vi "Driver - DTACQ - Get Detailed List of Commands.vi"(8 "error in":errorcluster, 11 "DTACQ Connection Data In":T1={"Description"="", "Address"="", "Port"=0, "timeout (ms)"=5000, "Termination Character"="\n", "TCP Connection Reference"=refnum, "Open Connection"=FALSE}) -> (0 "error out":errorcluster, 1 "Write Access":bool[](array[boolean]), 2 "Read Access":bool[](array[boolean]), 3 "DTACQ Connection Data Out":T1={"Description"="", "Address"="", "Port"=0, "timeout (ms)"=5000, "Termination Character"="\n", "TCP Connection Reference"=refnum, "Open Connection"=FALSE}, 4 "Command Descriptions":string[](array[string]), 5 "Commands":string[](array[string]))   [LabVIEW 2017, in "Communications Library.lvlib"]
doc: "Runs the help command2 and retrieves the response.\nEach command is outputted as an element of the command array.\nThe commands are ordered in the same order in which they are read from the DTACQ device.\n\nNote: the help2 command does not always produce a complete list of all possible commands. Only the commands where detailed help is availabe are included in the list."
uses:
  Communications Library.lvlib
  Typedefs/DTACQ Connection Data--Cluster.ctl
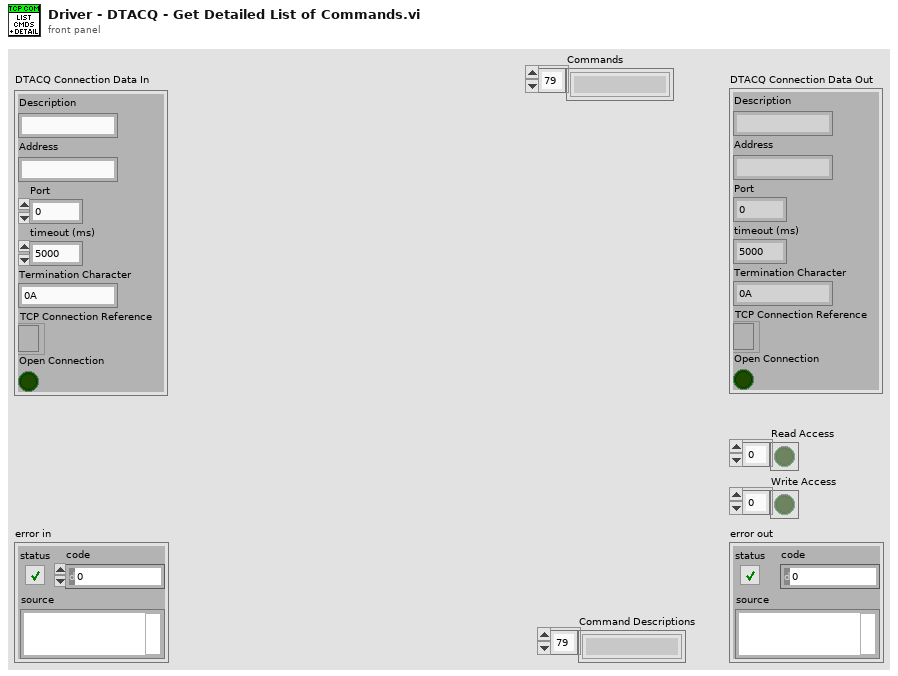
[diagram p1: front panel]
types:
  T1 = typedef "Communications Library.lvlib/DTACQ Connection Data--Cluster.ctl" = cluster{"Description":string, "Address":string, "Port":u16, "timeout (ms)":i32, "Termination Character":string, "TCP Connection Reference":refnum<k5>, "Open Connection":bool}
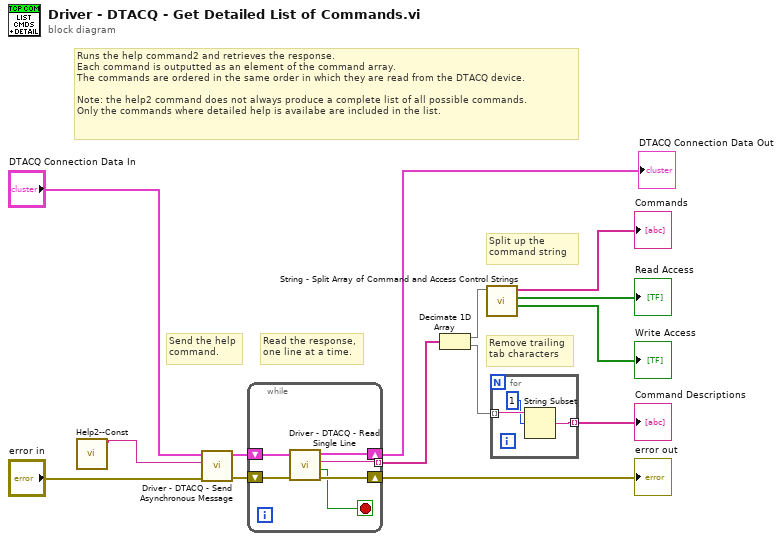
[diagram p0: block diagram]
diagram:
  # "Read the response,\none line at a time."
  # "Send the help\ncommand."
  # "Runs the help command2 and retrieves the response.\nEach command is outputted as an element of the command array.\nThe commands are ordered in the same order in which they are read from the DTACQ device.\n\nNote: the help2 command does not always produce a complete list of all possible commands.  \nOnly the commands where detailed help is availabe are included in the list."
  # "Split up the \ncommand string"
  # "Remove trailing\ntab characters"
  n1 = call "Help2--Const.vi"() -> ("Help2 Command"=w6:string)  [unwired: 11 in]
  n2 = call "Driver - DTACQ - Send Asynchronous Message.vi"("error in"="error in", "Message to Send"=w6, "DTACQ Connection Data In"="DTACQ Connection Data In") -> ("error out"=w8:errorcluster, "DTACQ Connection Data Out"=w7:T1)  [unwired: 7 in]
  n3 = while {
    shift-right: [w16] -> w2
    shift-left: w7 -> [w19]
    shift-right: [w18] -> w1
    shift-left: w8 -> [w20]
    tunnel: [w15] -> w3 mode=indexing
    stop <- w17 stop-if-true
    n4 = call "Driver - DTACQ - Read Single Line.vi"("error in"=w20, "DTACQ Connection Data In"=w19) -> ("error out"=w18:errorcluster, "Timed Out"=w17:bool, "Read String"=w15:string, "DTACQ Connection Data Out"=w16:T1)  [unwired: 6 in]
  }
  "error out" <- w1
  "DTACQ Connection Data Out" <- w2
  n5 = Decimate 1D Array(w3) -> (w14:string[], w10:string[])
  n6 = call "String - Split Array of Command and Access Control Strings.vi"("Commands and RW Properties"=w14) -> ("Write Access"=→"Write Access":bool[], "Read Access"=→"Read Access":bool[], "Commands"=→"Commands":string[])  [unwired: 8 in]
  n7 = for {
    tunnel: w10 -> [w23] mode=indexing
    tunnel: [w22] -> w9 mode=indexing
    n8 = String Subset(string=w23, offset (0)=1) -> (substring=w22:string)  [unwired: 1 in]
  }
  "Command Descriptions" <- w9
